vi "IntakeStateController.vi"(0 "Selected State (In)":string) -> ()   [LabVIEW 2019]
uses:
  dsinstructions.vi
  outputs.vi
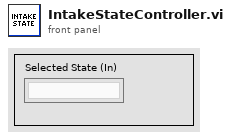
[diagram p1: front panel]
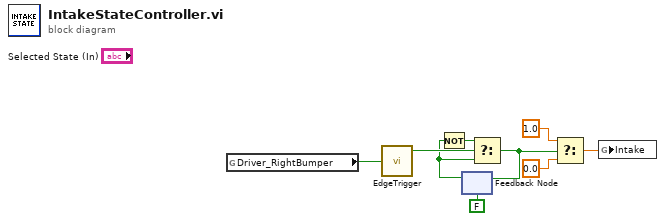
[diagram p0: block diagram]
diagram:
  n1 = global read "dsinstructions.vi" "Driver_RightBumper"() -> (w9:bool)
  n2 = call "EdgeTrigger.vi"("Input Signal"=w9) -> ("Rising Edge Trigger"=w8:bool)  [unwired: 2 out]
  n3 = feedback #1(FALSE ("Intake_On")) -> (w6:bool)
  n4 = Not(x=w6) -> (.not. x?=w5:bool)
  n5 = Select(t=w5, s=w8, f=w6) -> (s? t:f=w4:bool)
  n6 = feedback-in #1(w4) -> ()
  n7 = Select(t=1.0, s=w4, f=0.0) -> (s? t:f=w1:dbl)
  n8 = global write "outputs.vi" "Intake"(w1) -> ()
